vi "Main.vi"() -> ()   [LabVIEW 2016]
doc: "The roboRIO Project template acquires acceleration data from the onboard accelerometer and displays the changes of acceleration values in a waveform chart."
uses:
  <vilib>/myRIO/Instrument Drivers/Onboard IO/DIO/typedefs/DIO Reference.ctl
  <vilib>/myRIO/Common/Instrument Driver Framework/Utilities/typedefs/myRIO Generic Hardware Reference.ctl
  <vilib>/myRIO/Common/Instrument Driver Framework/Utilities/typedefs/Hardware Version Enum.ctl
  <vilib>/myRIO/Common/Instrument Driver Framework/Utilities/typedefs/myRIO v1.0 Reference.ctl
  <vilib>/myRIO/Common/Instrument Driver Framework/Utilities/typedefs/Generic FPGA Reference.ctl
  <vilib>/myRIO/Common/Instrument Driver Framework/myRIO v1.0/DIO/typedefs/DIO Channels List.ctl
  <vilib>/myRIO/Common/Instrument Driver Framework/myRIO v1.0/DIO/typedefs/DIO Channels Enum.ctl
  <vilib>/userdefined/High Color/nirio_resource_hc.ctl
  <vilib>/Platform/TimedLoop/XDataNode/timing_clust.ctl
  <vilib>/Platform/TimedLoop/XDataNode/nitl_modes.ctl
  <vilib>/Platform/TimedLoop/XDataNode/wakeup.ctl
  <vilib>/myRIO/Common/Instrument Driver Framework/Utilities/vis/Is FPGA Ref Available.vi
  <vilib>/myRIO/Common/Instrument Driver Framework/roboRIO v1.0/DIO/vis/roboRIO v1.0 Open DIO.vi
  <vilib>/myRIO/Instrument Drivers/Onboard IO/DIO/vis/Write.vi
  <vilib>/myRIO/Common/Instrument Driver Framework/Utilities/vis/Validate Channels.vi
  <vilib>/myRIO/Common/Instrument Driver Framework/roboRIO v1.0/DIO/vis/roboRIO v1.0 Reserve DIO.vi
  <vilib>/myRIO/Common/Instrument Driver Framework/roboRIO v1.0/DIO/vis/roboRIO v1.0 Build MUX Configuration DIO.vi
  <vilib>/myRIO/Common/Instrument Driver Framework/roboRIO v1.0/Resource Manager/vis/roboRIO v1.0 Reserve Channel List.vi
  <vilib>/myRIO/Common/Instrument Driver Framework/roboRIO v1.0/Resource Manager/vis/roboRIO v1.0 Create Configuration List.vi
  <vilib>/myRIO/Common/Instrument Driver Framework/roboRIO v1.0/Resource Manager/vis/roboRIO v1.0 Reserve Channel.vi
  <vilib>/myRIO/Common/Instrument Driver Framework/roboRIO v1.0/Resource Manager/vis/roboRIO v1.0 Unreserve Channel.vi
  <vilib>/myRIO/Common/Instrument Driver Framework/roboRIO v1.0/Resource Manager/vis/roboRIO v1.0 Build Mutex Name.vi
  <vilib>/FPGAPlugInAG/roboRIO/niLvFpga_Open_roboRIO.vi
  <vilib>/rvi/interface/common/dynamic/niFpgaDynamicAddResources.vi
  <vilib>/FPGAPlugInAG/Dynamic/niLvFpga_Reset_Dynamic.vi
  <vilib>/Utility/VariantDataType/GetNumericInfo.vi
  <vilib>/Utility/error.llb/Error Cluster From Error Code.vi
  <vilib>/myRIO/Common/Instrument Driver Framework/roboRIO v1.0/roboRIO v1.0 Open.vi
  <vilib>/myRIO/Common/Instrument Driver Framework/Utilities/vis/IO Manager.vi
  <vilib>/myRIO/Common/Instrument Driver Framework/Utilities/vis/Configuration Manager.vi
  <vilib>/myRIO/Common/Instrument Driver Framework/roboRIO v1.0/Resource Manager/vis/roboRIO v1.0 Configure IO.vi
  <vilib>/myRIO/Common/Instrument Driver Framework/myRIO v1.0/myRIO v1.0 Close.vi
  <vilib>/myRIO/Common/Instrument Driver Framework/roboRIO v1.0/DIO/vis/roboRIO v1.0 Write DIO.vi
  <vilib>/FPGAPlugInAG/Dynamic/niLvFpga_Run_Dynamic.vi
  <vilib>/rvi/errors/niLvFpgaAdjustHostInterfaceError.vi
  <vilib>/rvi/interface/nirviOpenFPGA/nirviOpenFPGA.xnode
  FPGA Bitfiles/AutoBikeProject_FPGATarget_AutoBikeFPGA_EwzLm8KNttI.lvbitx
  <vilib>/rvi/interface/nirviMethod/nirviMethod.xnode
  <vilib>/myRIO/Express VI/Onboard Devices/LED/LED Express VI.xnode
  <vilib>/myRIO/Instrument Drivers/Onboard IO/DIO/vis/myRIO DIO Open.xnode
  <vilib>/rvi/interface/nirviReadWriteControl/nirviReadWriteControl.xnode
  <vilib>/platform/TimedLoop/XDataNode/XDataNode.xnode
  <vilib>/Platform/TimedLoop/XDataNode/XDNodeRunTimeDep.lvlib
  <vilib>/rvi/interface/Simulation/niFpgaSimulationCallBeginRW.vi
  NiFpgaLv.dll
  <vilib>/addons/Fuzzy Logic/NI_Fuzzy_Logic_API.lvlib
  <vilib>/myRIO/Instrument Drivers/Onboard IO/DIO/DIO.lvlib
panel:
  in  "Freq":dbl
  in  "Number of bias loops":i32=1000
  in  "Calc bias":bool
  in  "Stop Button":bool
  in  "Velocity reference":sgl=15.0
  in  "Front Panel Duty Cycle":dbl(slide) scale=0.0..1.0
  in  "error in (no error)":errorcluster
  in  "Front Panel Switch direction":bool
  out "Main loop lates":i32
  out "IMU loop lates":i32
  out "Duty cycle BW":sgl
  out "Stopping":bool
  out "Velocity chart":dbl(graph)
  out "error out fuzzy":errorcluster
  out "Roll & Pitch":cluster{"xAngle":dbl, "yAngle":dbl}(graph)
  out "IMU loop finished late":bool
  out "mA":dbl[](array[numeric])
  out "pitch":dbl
  out "roll":dbl
  out "Bias":T1
  out "error out IMU loop":errorcluster
  out "Current velocity":dbl
  out "Steering angle (degrees)":sgl
  out "error out main loop":errorcluster
  out "Main Loop finish late":bool
  # "INPUTS"
  # "OUTPUTS"
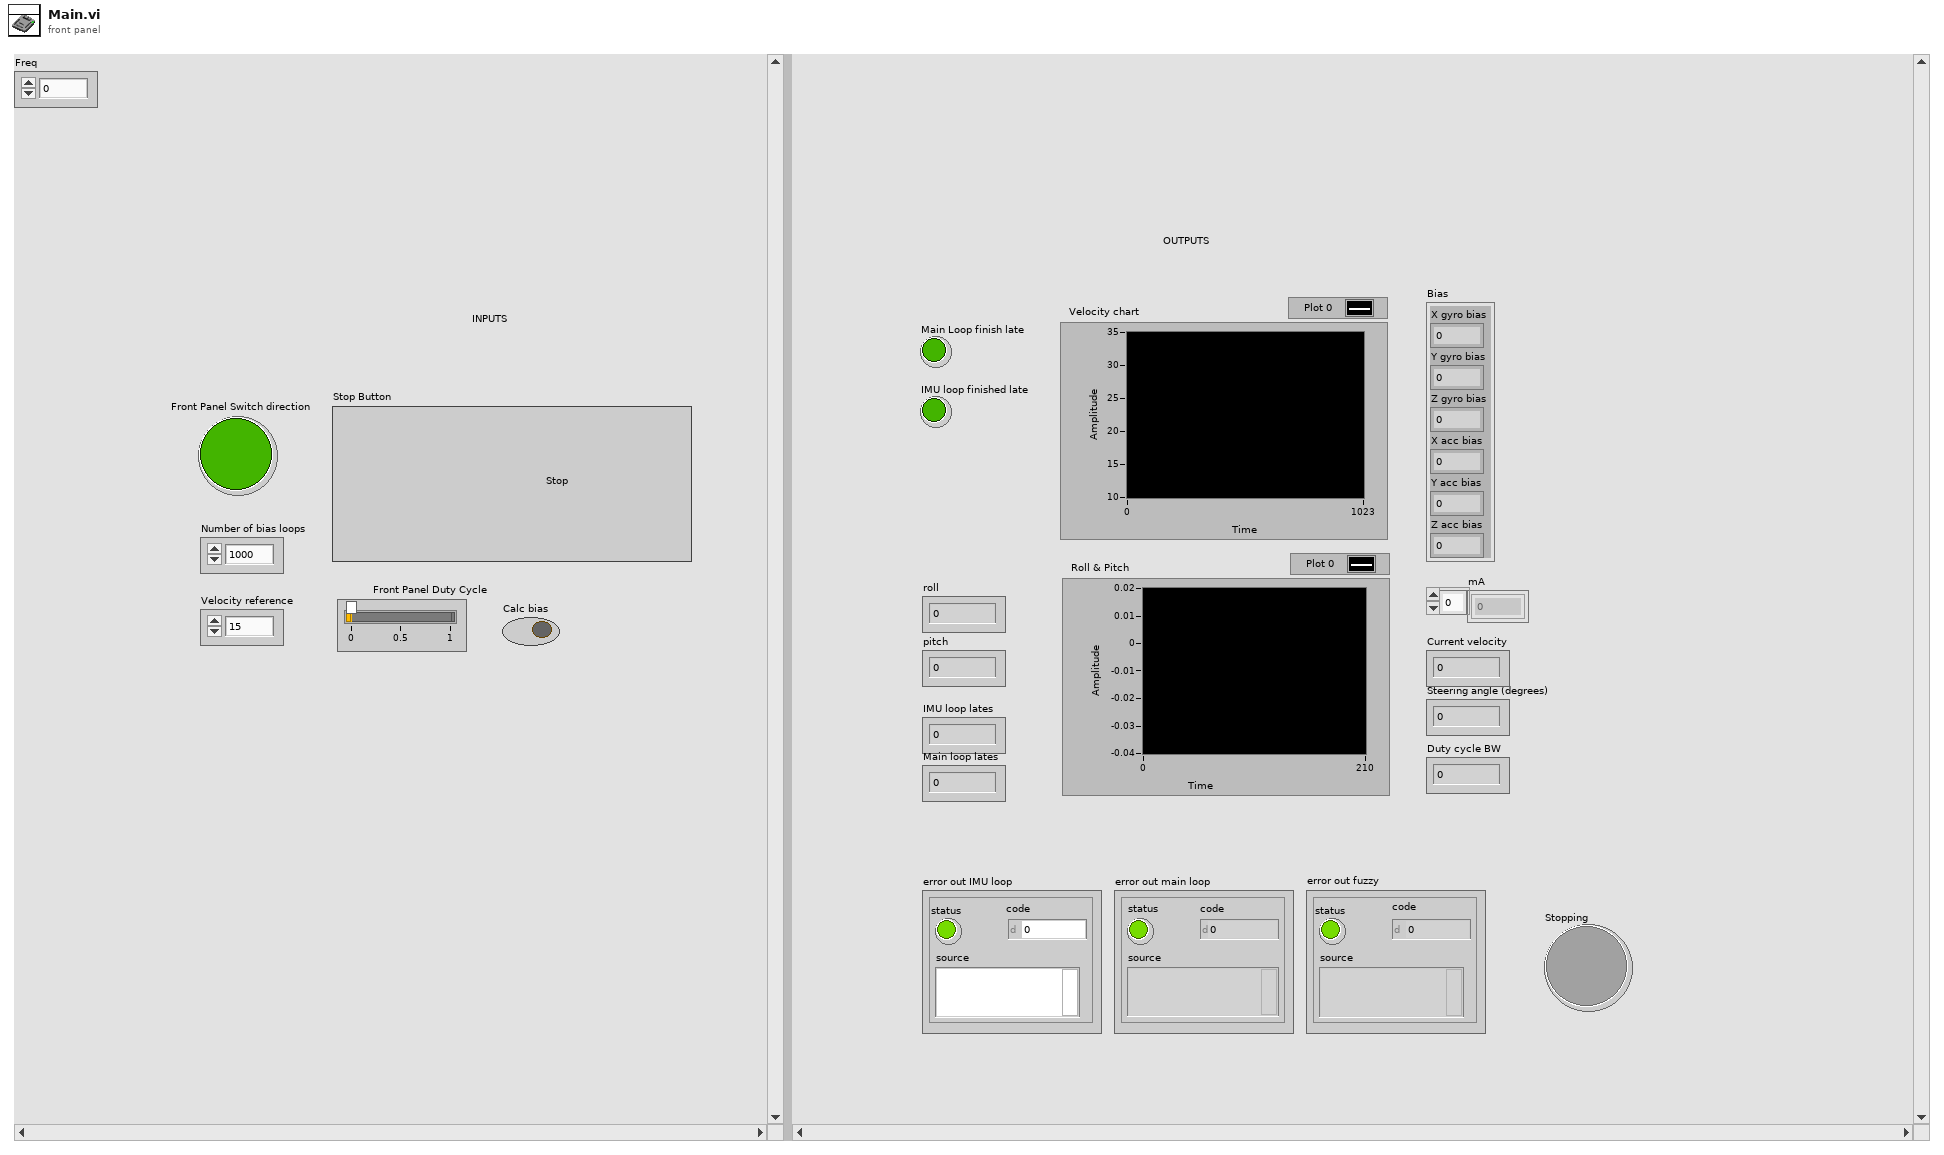
[diagram p1: front panel]
types:
  T1 = cluster{"X gyro bias":dbl, "Y gyro bias":dbl, "Z gyro bias":dbl, "X acc bias":dbl, "Y acc bias":dbl, "Z acc bias":dbl}
  T2 = typedef "DIO.lvlib/DIO Reference.ctl" = cluster{"myRIO Reference":T3, "DIO Channels List":T7}
  T3 = typedef "myRIO Generic Hardware Reference.ctl" = cluster{"myRIO Model":T4, "myRIO Hardware Reference":T5}
  T4 = typedef "Hardware Version Enum.ctl" = enum16{"Unknown", "myRIO-1900", "myRIO-1950", "roboRIO", "NI ELVIS RIO CM"}
  T5 = typedef "myRIO v1.0 Reference.ctl" = cluster{"Generic FPGA Reference":T6, "Allow multiple opens":bool}
  T6 = typedef "Generic FPGA Reference.ctl" = refnum<k20>
  T7 = typedef "DIO Channels List.ctl" = T8[]
  T8 = typedef "DIO Channels Enum.ctl" = enum16{"Not Connected", "C/DIO0", "C/DIO1", "C/DIO2", "C/DIO3", "C/DIO4", "C/DIO5", "C/DIO6", "C/DIO7", "A/DIO0", "A/DIO1", "A/DIO2", "A/DIO3", "A/DIO4", "A/DIO5", "A/DIO6", "A/DIO7", "A/DIO8", "A/DIO9", "A/DIO10", "A/DIO11", "A/DIO12", "A/DIO13", "A/DIO14", "A/DIO15", "B/DIO0", "B/DIO1", "B/DIO2", "B/DIO3", "B/DIO4", "B/DIO5", "B/DIO6", "B/DIO7", "B/DIO8", "B/DIO9", "B/DIO10", "B/DIO11", "B/DIO12", "B/DIO13", "B/DIO14", "B/DIO15", "LED0", "LED1", "LED2", "LED3", "Button0", "DIO/DIO0", "DIO/DIO1", "DIO/DIO2", "DIO/DIO3", "DIO/DIO4", "DIO/DIO5", "DIO/DIO6", "DIO/DIO7", "DIO/DIO8", "DIO/DIO9", "SPI/CS0", "SPI/CS1", "SPI/CS2", "SPI/CS3", "LED RADIO (Green)", "LED RADIO (Red)", "LED COMM (Green)", "LED COMM (Red)", "LED MODE (Green)", "LED MODE (Red)"}
  T9 = typedef "nirio_resource_hc.ctl" = tag
  T10 = typedef "XDNodeRunTimeDep.lvlib/timing_clust.ctl" = cluster{"Expected End [f-1]":u64, "Actual End [f-1]":u64, "Finished Late? [f-1]":bool, "Expected End [i-1]":u64, "Actual End [i-1]":u64, "Finished Late? [i-1]":bool, "Expected Start [i]":u64, "Actual Start [i]":u64, "Expected Start [f]":u64, "Actual Start [f]":u64, "Source Name":string, "Structure Name":string, "Period":i64, "Deadline":i64, "Offset":i64, "Start":i64, "Priority":i32, "Timeout":i32, "Mode":T11, "Wakeup Reason":T12, "Error":errorcluster, "Source Type":string, "Secondary Source Type":string, "Global End Time":u64, "Global Start Time":u64, "Frame Duration":u64, "Iteration Duration":u64, "Assigned CPU":i32, "I/O Scan Engine Mode":u32}
  T11 = typedef "XDNodeRunTimeDep.lvlib/nitl_modes.ctl" = enum32{"No Change", "Process missed periods, maintain original phase", "Discard missed periods, maintain original phase", "Process missed periods, ignore original phase", "Discard missed periods, ignore original phase"}
  T12 = typedef "XDNodeRunTimeDep.lvlib/wakeup.ctl" = enum32{"Normal", "Aborted", "Asynchronous wakeup", "Timing source error", "Timed loop error", "Timeout"}
  T13 = typedef "NI_Fuzzy_Logic_API.lvlib/FL System.ctl" = cluster{"input variables":T14[], "output variables":T14[], "rules":T17[], "defuzzification method":T23, "description":string, "user MF interpolating polynomials":T24[]}
  T14 = typedef "NI_Fuzzy_Logic_API.lvlib/FL Variable.ctl" = cluster{"name":string, "range":dbl[], "MFs":T15[]}
  T15 = typedef "NI_Fuzzy_Logic_API.lvlib/FL Membership Function.ctl" = cluster{"name":string, "shape":T16, "points":dbl[], "color":u32, "user-defined shape index":i32}
  T16 = typedef "NI_Fuzzy_Logic_API.lvlib/FL Membership Function Shape.ctl" = u16
  T17 = typedef "NI_Fuzzy_Logic_API.lvlib/FL Rule.ctl" = cluster{"antecedents":T18[], "antecedent connective":T20, "consequents":T21[], "consequent implication":T22, "degree of support":dbl}
  T18 = typedef "NI_Fuzzy_Logic_API.lvlib/FL Antecedent.ctl" = cluster{"Var Index":i32, "MF Index":i32, "Cond":T19}
  T19 = typedef "NI_Fuzzy_Logic_API.lvlib/FL Modifier.ctl" = u16
  T20 = typedef "NI_Fuzzy_Logic_API.lvlib/FL Antecedent Connective.ctl" = u16
  T21 = typedef "NI_Fuzzy_Logic_API.lvlib/FL Consequent.ctl" = cluster{"Var Index":i32, "MF Index":i32, "Cond":T19}
  T22 = typedef "NI_Fuzzy_Logic_API.lvlib/FL Consequent Implication.ctl" = u16
  T23 = typedef "NI_Fuzzy_Logic_API.lvlib/FL Defuzzification.ctl" = u16
  T24 = typedef "NI_Fuzzy_Logic_API.lvlib/FL Interpolating polynomials.ctl" = cluster{"X":dbl[], "Y":dbl[], "Y(x) coeff":dbl[][], "X(y) coeff":dbl[][], "Area(y) coeff":dbl[][], "coa_x(y) coeff":dbl[][]}
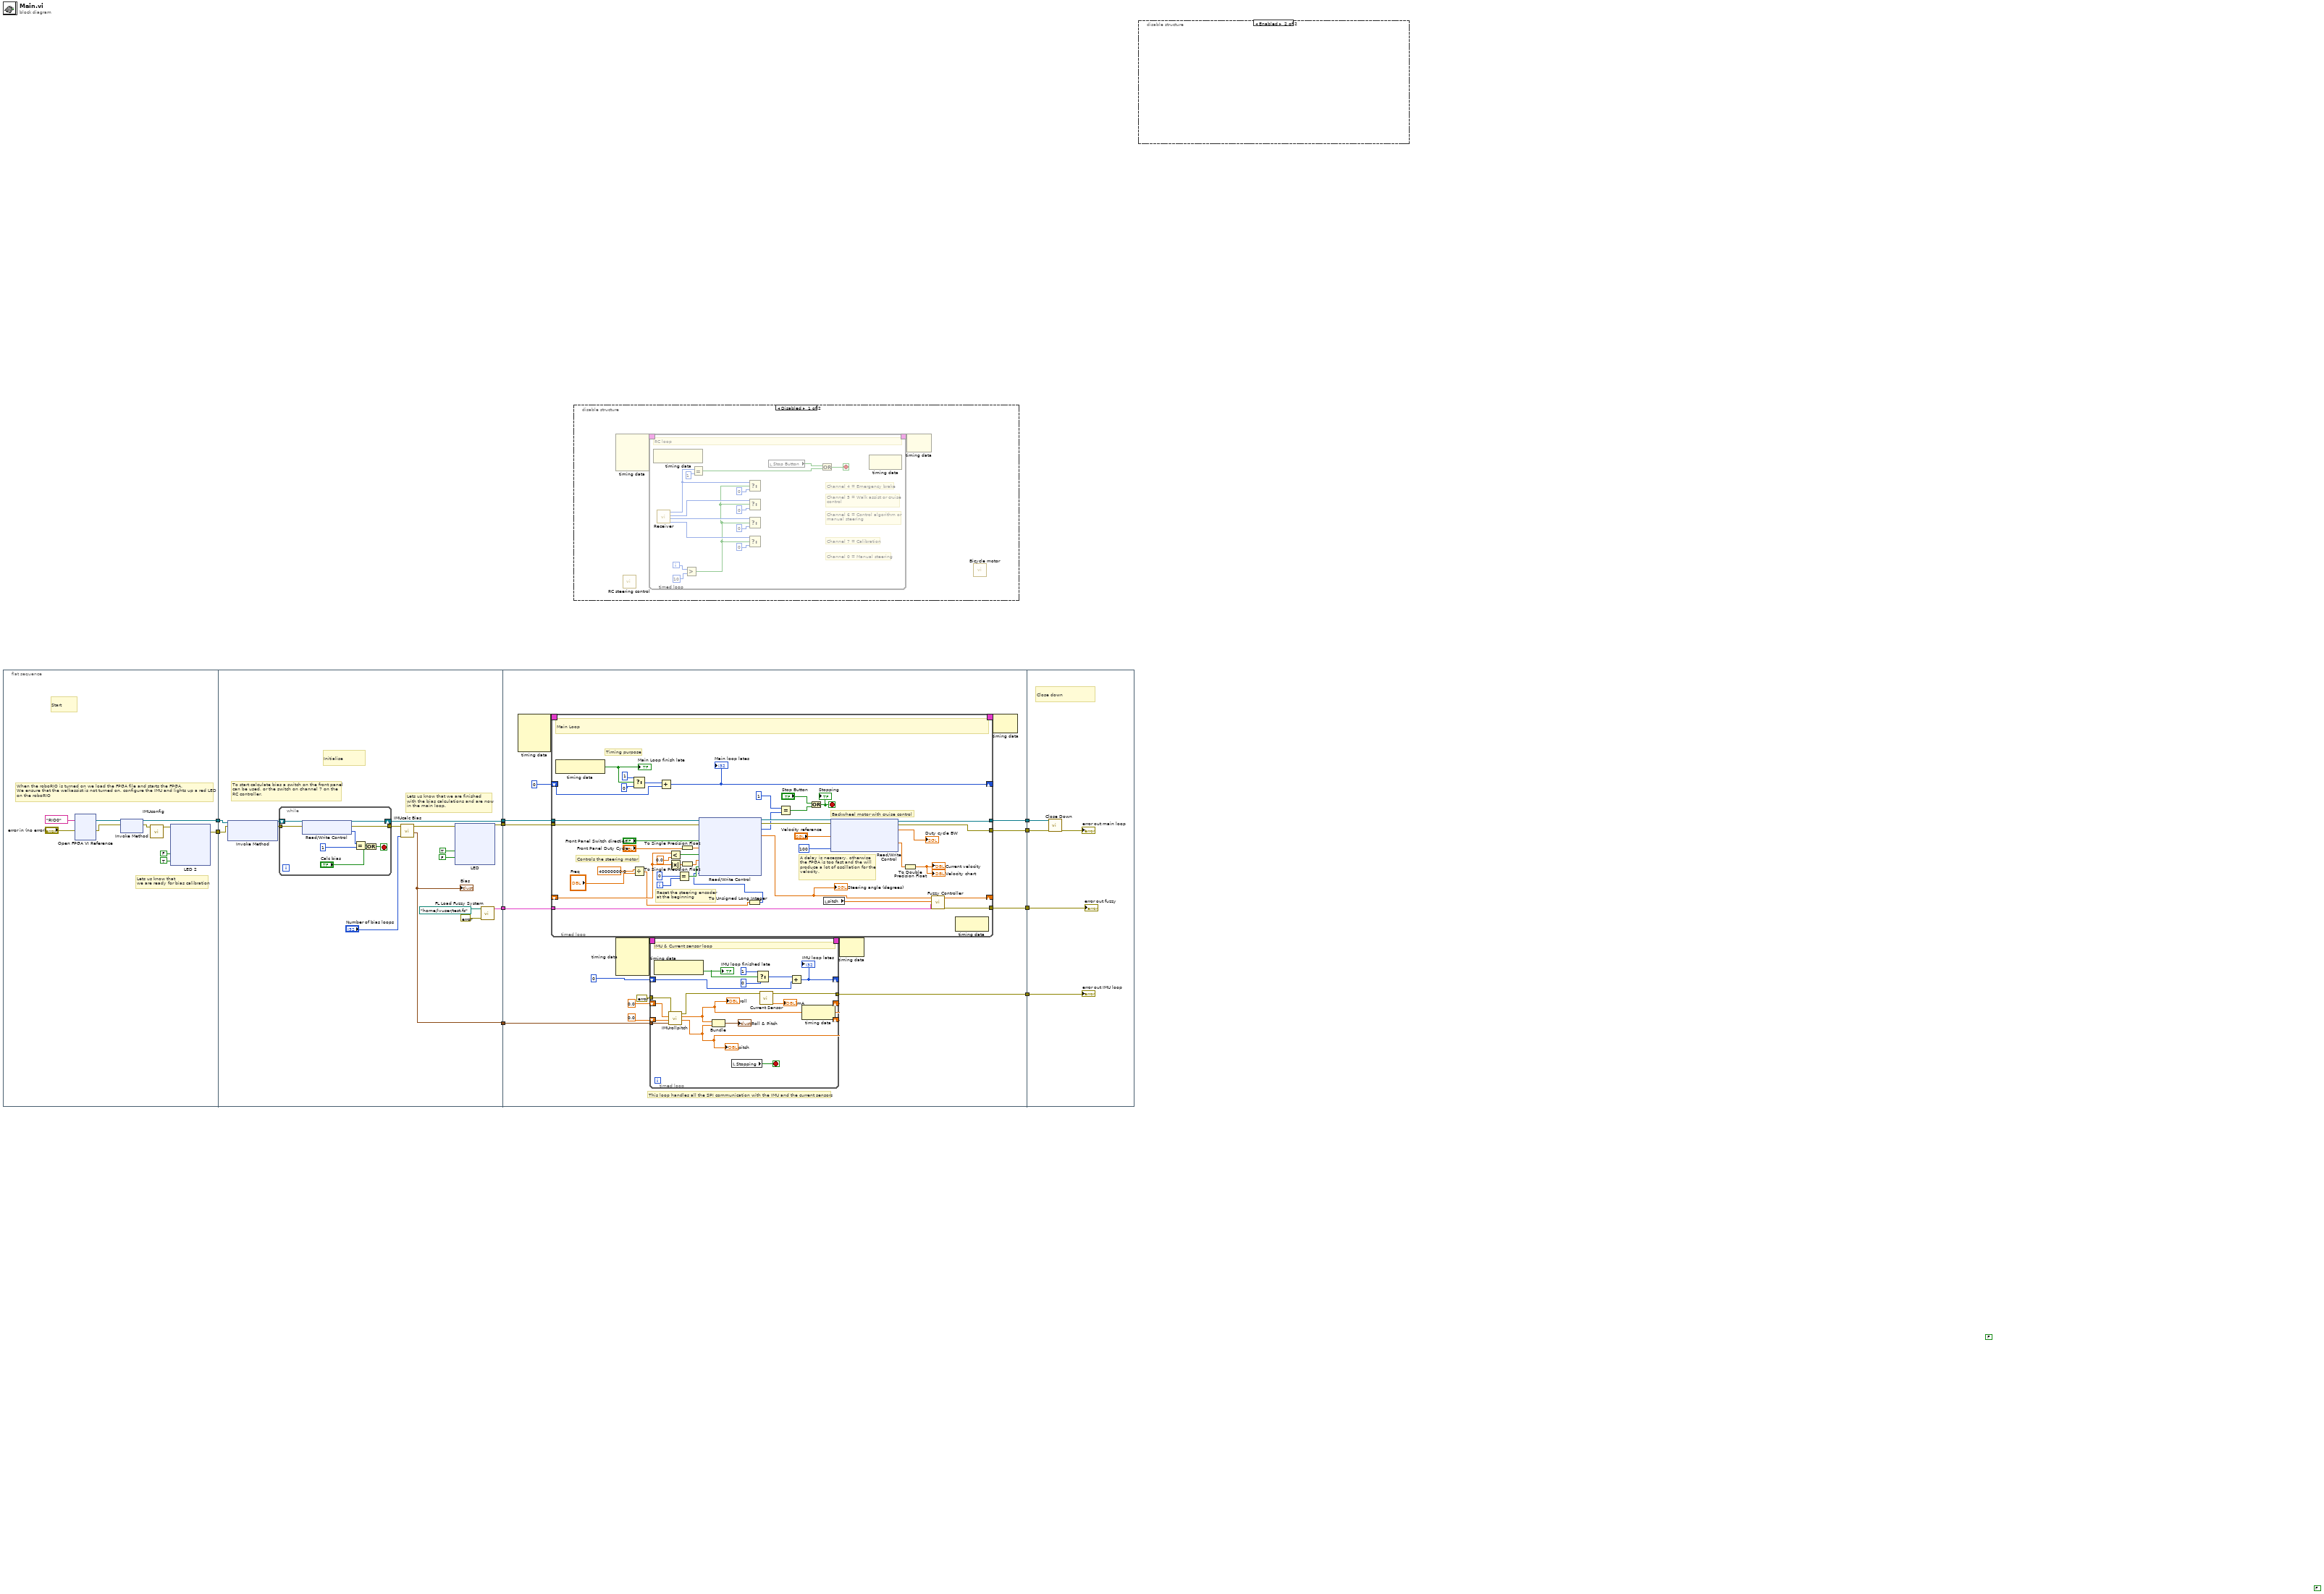
[diagram p0: block diagram]
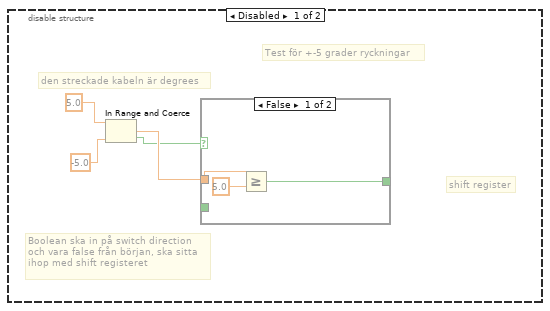
[diagram p3: hidden frame]
diagram:
  (unwired) FALSE
  (unwired) FALSE
  n1 = flat-sequence {
    tunnel: [w13] -> w4
    tunnel: [w12] -> w3
    tunnel: [w60] -> w10
    tunnel: [w64] -> w9
    tunnel: [w71] -> w8
    tunnel: w4 -> [w63]
    tunnel: w3 -> [w57]
    tunnel: [w67] -> w5
    tunnel: w10 -> [w132]
    tunnel: w9 -> [w133]
    tunnel: [w131] -> w7
    tunnel: [w130] -> w6
    tunnel: w8 -> [w127]
    tunnel: w5 -> [w121]
    tunnel: [w120] -> w2
    tunnel: [w119] -> w1
    tunnel: w7 -> [w203]
    tunnel: w6 -> [w207]
    tunnel: w2 -> [w205]
    tunnel: w1 -> [w204]
    frame #0 {
      # "Start"
      # "Lets us know that\nwe are ready for bias calibration"
      # "When the roboRIO is turned on we load the FPGA file and starts the FPGA.\nWe ensure that the walkassist is not turned on, configure the IMU and lights up a red LED\non the roboRIO"
      n2 = xnode "Open FPGA VI Reference"("error in"="error in (no error)", "resource name"=tag "RIO0") -> ("FPGA VI Reference Out"=w19:refnum<k20>, "error out"=w20:errorcluster)
      n3 = xnode "Invoke Method"("FPGA VI Reference In"=w19, "error in"=w20) -> ("FPGA VI Reference Out"=w12:refnum<k20>, "error out"=w11:errorcluster)
      n4 = call "IMUconfig.vi"("error in (no error)"=w11) -> ("error out"=w14:errorcluster)  [unwired: 10 in]
      n5 = xnode "LED 2"("COMM (Green)"=FALSE, "COMM (Red)"=TRUE, "error in (no error)"=w14) -> ("error out"=w13:errorcluster)
    }
    frame #1 {
      # "Lets us know that we are finished\nwith the bias calculations and are now\nin the main loop."
      # "To start calculate bias a switch on the front panel\ncan be used, or the switch on channel 7 on the \nRC controller."
      # "Initialise"
      n6 = xnode "Invoke Method"("FPGA VI Reference In"=w57, "error in"=w63) -> ("FPGA VI Reference Out"=w62:refnum<k20>, "error out"=w61:errorcluster)  [unwired: 1 in]
      n7 = while {
        tunnel: w61 -> [w79]
        shift-right: [w78] -> w60
        shift-left: w62 -> [w80]
        tunnel: [w77] -> w59
        stop <- w73 stop-if-true
        n8 = xnode "Read/Write Control"("FPGA VI Reference In"=w80, "error in"=w79) -> ("FPGA VI Reference Out"=w78:refnum<k20>, "error out"=w77:errorcluster, "Channel 7 position"=w76:i32)
        n9 = Equal?(x=w76, y=1) -> (x = y?=w74:bool)
        n10 = Or(x=w74, y="Calc bias") -> (x .or. y?=w73:bool)
      }
      n11 = call "IMUcalc Bias.vi"("Number of loops"="Number of bias loops", "error in (no error)"=w59) -> ("Bias"=w71:T1, "error out"=w58:errorcluster)  [unwired: 7 in]
      "Bias" <- w71
      n12 = xnode "LED"("COMM (Green)"=TRUE, "COMM (Red)"=FALSE, "error in (no error)"=w58) -> ("error out"=w64:errorcluster)
      n13 = call <vilib>:"FL Load Fuzzy System.vi"("error in (no error)"=errorcluster {"status"=FALSE, "code"=0, "source"=""}, "file path"=path "/home/lvuser/test.fs") -> ("fuzzy system out"=w67:T13)  [unwired: 8 in, 1 out]
    }
    frame #2 {
      # "This loop handles all the SPI communication with the IMU and the current sensors"
      n14 = node-c288() -> (w123:T10)  [unwired: 4 in]
      n15 = timed-loop {
        timing: w123 -> [_]
        timing-out: [_] -> w122
        tunnel: w133 -> [w162]
        tunnel: [w173] -> w131
        tunnel: w132 -> [w163]
        tunnel: [w138] -> w130
        tunnel: w121 -> [w169]
        tunnel: [w168] -> w119
        shift-right: [w167] -> _
        shift-left: _ -> [w165]
        shift-right: [w141] -> _
        shift-left: 0 -> [w140]
        i -> [w174]
        stop <- w170 stop-if-true
        # "Reset the steering encoder\nat the beginning"
        # "A delay is necessary, otherwise \nthe FPGA is too fast and the will \nproduce a lot of oscillation for the\nvelocity."
        # "Controls the steering motor"
        # "Backwheel motor with cruise control"
        # "Timing purpose"
        # "Main Loop"
        n16 = node-c288() -> (w145:bool)  [unwired: 1 in]
        "Main Loop finish late" <- w145
        n17 = Select(t=1, s=w145, f=0) -> (s? t:f=w143:i32)
        n18 = Divide(x=40000000.0, y="Freq") -> (x/y=w134:dbl)
        n19 = Add(x=w143, y=w140) -> (x+y=w141:i32)
        "Main loop lates" <- w141
        n20 = Less?(x=w165, y=0.0) -> (x < y?=w151:bool)
        n21 = Absolute Value(x=w165) -> (abs(x)=w150:dbl)
        n22 = Equal?(x=0, y=w174) -> (x = y?=w147:bool)
        n23 = To Single Precision Float(number="Front Panel Duty Cycle") -> (single precision float=w153:sgl)
        n24 = To Single Precision Float(number=w150) -> (single precision float=w149:sgl)
        n25 = To Unsigned Long Integer(number=w134) -> (unsigned 32bit integer=w135:u32)
        n26 = xnode "Read/Write Control"("FPGA VI Reference In"=w163, "error in"=w162, "Front Panel Direction"="Front Panel Switch direction", "Front Panel Duty Cycle"=w153, "Control Loop Direction"=w151, "Control Loop Duty Cycle"=w149, "Reset counter"=w147, "Freq"=w135) -> ("FPGA VI Reference Out"=w157:refnum<k20>, "error out"=w156:errorcluster, "Channel 4 position"=w146:i32, "Steering angle(deg)"=w148:sgl)
        "Steering angle (degrees)" <- w148
        n27 = Equal?(x=1 ("y"), y=w146) -> (x = y?=w172:bool)
        n28 = Or(x="Stop Button", y=w172) -> (x .or. y?=w170:bool)
        "Stopping" <- w170
        n29 = local read "pitch"() -> (w164:dbl)
        n30 = xnode "Read/Write Control"("FPGA VI Reference In"=w157, "error in"=w156, "Reference velocity in km/h"="Velocity reference", "Count(uSec)"=u32 100) -> ("FPGA VI Reference Out"=w173:refnum<k20>, "error out"=w138:errorcluster, "Duty cycle (BW)"=→"Duty cycle BW":sgl, "Current velocity"=w160:sgl)
        n31 = To Double Precision Float(number=w160) -> (double precision float=→"Current velocity" →"Velocity chart":dbl)
        n32 = call "Fuzzy Controller.vi"("fuzzy system in"=w169, "pitch"=w164, "Steering angle(deg)"=w148) -> ("error out"=w168:errorcluster, "output value"=w167:dbl)  [unwired: 7 in]
        n33 = node-c288() -> ()  [unwired: 1 in, 1 out]
      }
      n34 = node-c288() -> (w129:T10)  [unwired: 4 in]
      n35 = timed-loop {
        timing: w129 -> [_]
        timing-out: [_] -> w128
        tunnel: w127 -> [w197]
        tunnel: errorcluster {"status"=FALSE, "code"=0, "source"=""} ("error in (no error)") -> [w194]
        shift-right: [w193] -> _
        shift-left: 0.0 ("xAngle in") -> [w196]
        shift-right: [w192] -> _
        shift-left: 0.0 ("xAngle in") -> [w195]
        tunnel: [w188] -> w120
        shift-right: [w182] -> _
        shift-left: 0 ("t") -> [w181]
        stop <- w187 stop-if-true
        # "IMU & Current sensor loop"
        n36 = node-c288() -> (w186:bool)  [unwired: 1 in]
        "IMU loop finished late" <- w186
        n37 = call "IMUrollpitch.vi"("Bias"=w197, "yAngle in"=w195, "xAngle in"=w196, "error in (no error)"=w194) -> ("pitch"=w192:dbl, "roll"=w193:dbl, "error out"=w189:errorcluster)  [unwired: 3 in, 2 out]
        "roll" <- w193
        "pitch" <- w192
        n38 = Bundle("roll"=w193, "pitch"=w192) -> (→"Roll & Pitch":cluster{"roll":dbl, "pitch":dbl})  [unwired: 1 in]
        n39 = local read "Stopping"() -> (w187:bool)
        n40 = Select(t=1, s=w186, f=0 ("t")) -> (s? t:f=w183:i32)
        n41 = call "Current Sensor.vi"("error in (no error)"=w189) -> ("mA"=→"mA":dbl[], "error out"=w188:errorcluster)  [unwired: 9 in]
        n42 = Add(x=w183, y=w181) -> (x+y=w182:i32)
        "IMU loop lates" <- w182
        n43 = node-c288() -> ()  [unwired: 1 in, 1 out]
      }
      n44 = node-c288(w128) -> ()  [unwired: 1 out]
      n45 = node-c288(w122) -> ()  [unwired: 1 out]
    }
    frame #3 {
      # "Close down"
      n46 = call "Close Down.vi"("error in (no error)"=w207, "FPGA VI Reference Out 2"=w203) -> ("error out"=→"error out main loop":errorcluster)  [unwired: 9 in]
      "error out fuzzy" <- w204
      "error out IMU loop" <- w205
    }
  }
  n47 = disable-structure shown="Disabled" {
    frame Disabled {
      n48 = node-c288() -> (w209:T10)  [unwired: 4 in]
      n49 = call "RC steering control.vi"() -> ()  [unwired: 10 in, 2 out]
      n50 = timed-loop {
        timing: w209 -> [_]
        timing-out: [_] -> w208
        i -> [w212]
        stop <- w225 stop-if-true
        # "Channel 7 = Calibration"
        # "Channel 0 = Manual steering"
        # "Channel 6 = Control algorithm or\nmanual steering"
        # "Channel 5 = Walk assist or cruise\ncontrol"
        # "Channel 4 = Emergency brake"
        # "RC loop"
        n51 = node-c288() -> (w229:bool)  [unwired: 1 in]
        n52 = call "Receiver.vi"() -> ("Channel 7 position"=w220:i32, "Channel 6 position"=w221:i32, "Channel 5 position"=w222:i32, "Channel 4 position"=w224:i32, 4:w230)  [unwired: 7 in]
        n53 = Greater?(x=w212, y=10) -> (0:w210:bool)
        n54 = Equal?(x=w224, y=1) -> (x = y?=w227:bool)
        n55 = Select(t=w224, s=w210, f=0) -> (s? t:f=w223:i32)
        n56 = Select(t=w222, s=w210, f=0) -> (s? t:f=w215:i32)
        n57 = Select(t=w221, s=w210, f=0) -> (s? t:f=w214:i32)
        n58 = Select(t=w220, s=w210, f=0) -> (s? t:f=w213:i32)
        n59 = local read "Stop Button"() -> (w228:bool)
        n60 = Or(x=w228, y=w227) -> (x .or. y?=w225:bool)
        n61 = node-c288() -> ()  [unwired: 1 in, 1 out]
      }
      n62 = node-c288(w208) -> ()  [unwired: 1 out]
      n63 = call "Bicycle motor.vi"() -> ()  [unwired: 8 in, 4 out]
    }
    frame Enabled {
    }
  }
  n64 = disable-structure shown="Enabled" {
    frame Disabled {
      # "Test för +-5 grader ryckningar"
      # "den streckade kabeln är degrees"
      # "Boolean ska in på switch direction\noch vara false från början, ska sitta\nihop med shift registeret"
      # "shift register"
      n65 = In Range and Coerce(upper limit=5.0, lower limit=-5.0) -> (x=w239:dbl, In Range?=w238:bool)  [unwired: 1 out]
      n66 = case shown="False" w238 {
        tunnel: w239 -> [w242 _]
        tunnel: [w240 w243] -> _
        tunnel: _ -> [_ w243]
        frame False {
          n67 = Greater Or Equal?(x=w242, y=5.0) -> (x >= y?=w240:bool)
        }
        frame True {
        }
      }
    }
    frame Enabled {
    }
  }
